vi "sv_Waterfall Display for Octave.vi"() -> ()   [LabVIEW 2017]
uses:
  <vilib>/addons/Sound and Vibration/compatibility/Waterfall/subVIs/sv_Waterfall for Octave Global.vi
panel:
  in  "palette":T1={"x axis width [%]"=80.0, "z axis height [%]"=40.0, "autoscale x"=FALSE, "autoscale y"=FALSE, "autoscale z max"=FALSE, "autoscale all"=FALSE, "transparency"=FALSE, "store view"=FALSE, "restore view"=FALSE} {"x axis width [%]" min=10.0 max=100.0 step=1.0 scale=10.0..100.0 scale format="%.1f"; "z axis height [%]" min=10.0 max=99.99 step=1.0 scale=10.0..100.0 scale format="%.1f"}
  in  "stop":bool
  in  "y axis":dbl(slide)=1234.0 scale=0.0..2.0 scale format="%.1f"
  in  "z axis":dbl(slide) scale=0.0..90.0 scale format="%.1f"
  in  "x axis":dbl(slide) scale=10.0..10000.0 scale format="%.1f"
  out "Graph":cluster{dbl[], dbl[]}[](graph)
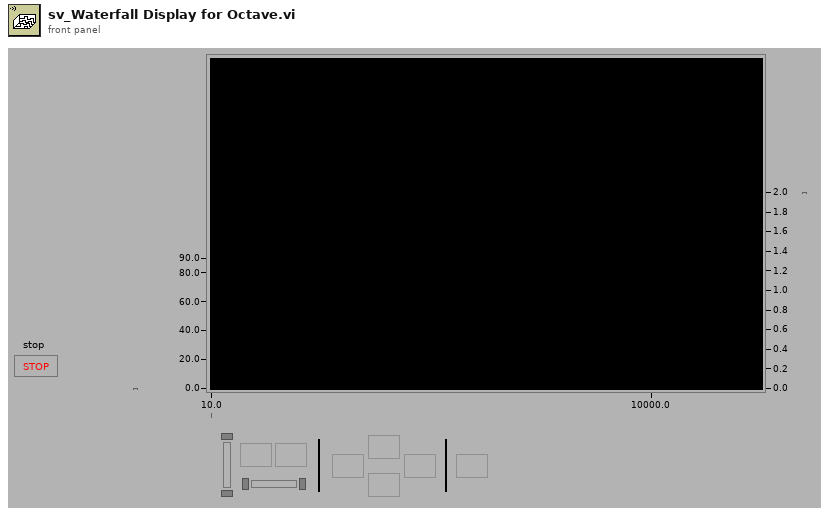
[diagram p1: front panel]
types:
  T1 = cluster{"x axis width [%]":dbl, "z axis height [%]":dbl, "autoscale x":bool, "autoscale y":bool, "autoscale z max":bool, "autoscale all":bool, "transparency":bool, "store view":bool, "restore view":bool}
  T2 = cluster{"autoscale x":bool, "autoscale y":bool, "autoscale z":bool, "autoscale all":bool, "transparency":bool, "store view":bool, "restore view":bool}
  T3 = cluster{"x axis width [%]":dbl, "z axis height [%]":dbl, "x axis minimum":dbl, "x axis maximum":dbl, "z axis minimum":dbl, "z axis maximum":dbl, "y axis minimum":dbl, "y axis maximum":dbl}
  T4 = typedef "LVPositionTypeDef.ctl" = cluster{"Left":i32, "Top":i32}
  T5 = cluster{"f low":dbl, "f high":dbl, "midband":dbl}[]
  T6 = cluster{"x axis width [%]":dbl, "z axis height [%]":dbl, "Scale.Minimum":dbl, "Scale.Maximum":dbl, "Scale.Minimum":dbl, "Scale.Maximum":dbl, "Scale.Minimum":dbl, "Scale.Maximum":dbl}
  T7 = cluster{"autoscale x":bool, "autoscale y":bool, "autoscale z max":bool, "autoscale all":bool, "transparency":bool, "store view":bool, "restore view":bool}
  T8 = cluster{"x axis width [%]":bool, "z axis height [%]":bool, bool, bool, bool, bool, bool, bool}
  T9 = cluster{"autoscale x":bool, "autoscale y":bool, bool, "autoscale all":bool, "transparency":bool, "store view":bool, "restore view":bool}
  T10 = cluster{bool, "x axis width [%]":dbl, "z axis height [%]":dbl, "Scale.Minimum":dbl, "Scale.Maximum":dbl, "Scale.Minimum":dbl, "Scale.Maximum":dbl, "Scale.Minimum":dbl, "Scale.Maximum":dbl, "transparency":bool}
  T11 = cluster{"x axis":string, "y axis":string, "z axis":string}
  T12 = cluster{"Scale.Minimum":dbl, "Scale.Maximum":dbl}
  T13 = cluster{"y index":i32, "y length":i32, "x index":i32, "x length":i32}
  T14 = cluster{"frame":u32, "plot":u32, "background":u32}
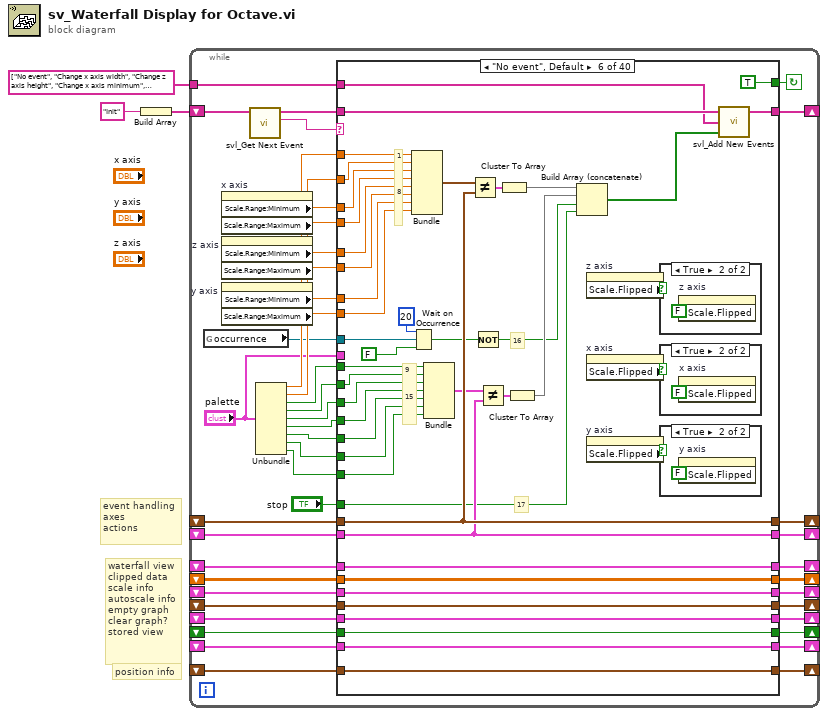
[diagram p0: block diagram]
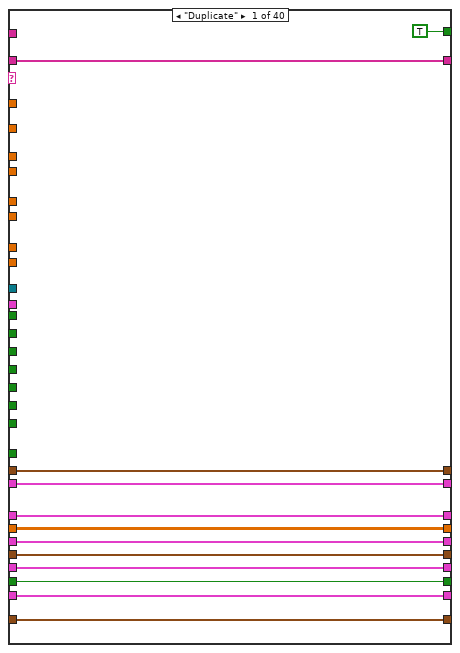
[diagram p2: hidden frame]
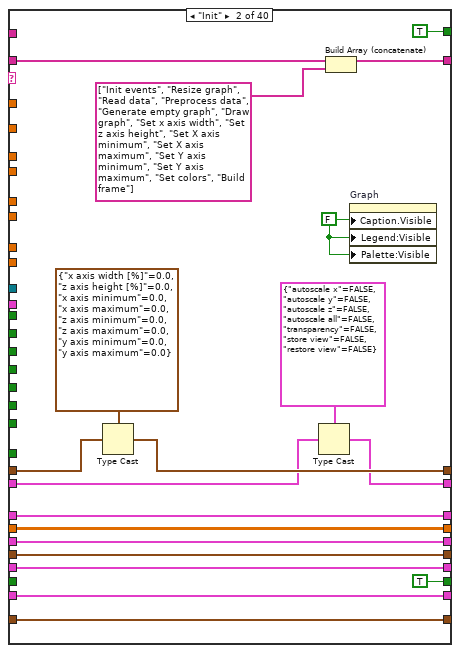
[diagram p3: hidden frame]
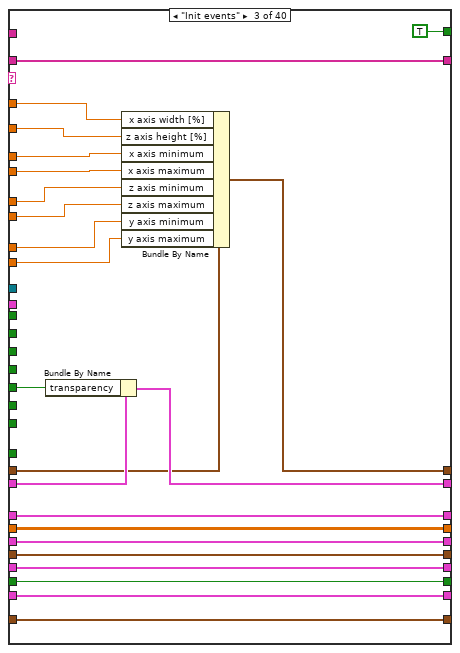
[diagram p4: hidden frame]
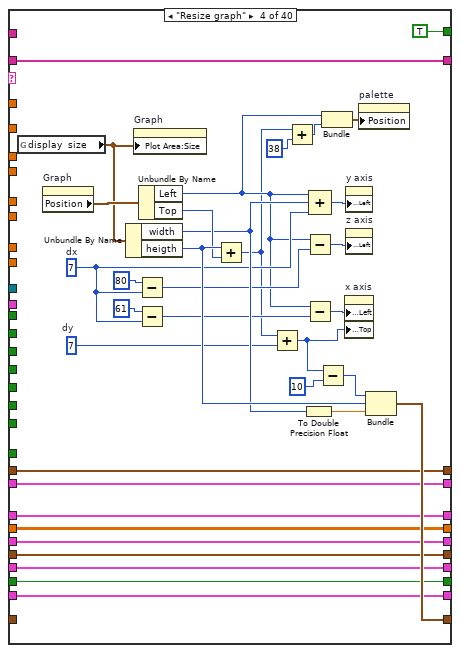
[diagram p5: hidden frame]
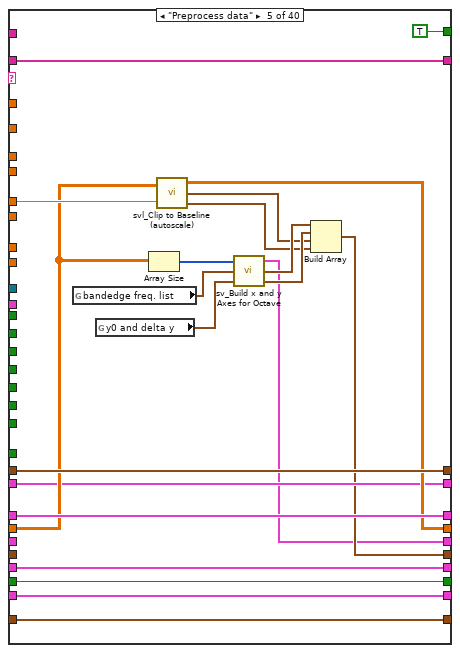
[diagram p6: hidden frame]
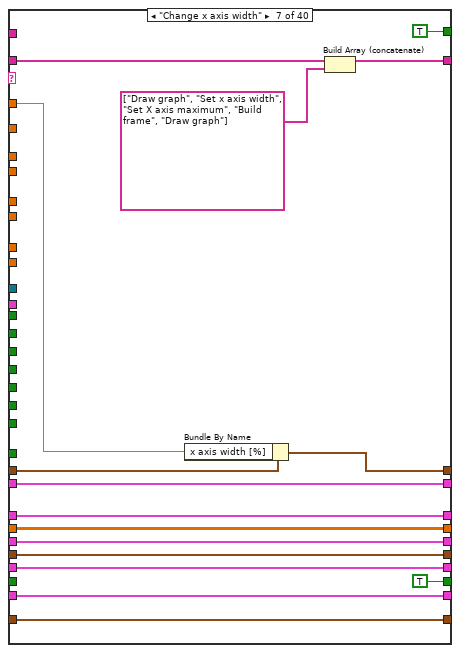
[diagram p10: hidden frame]
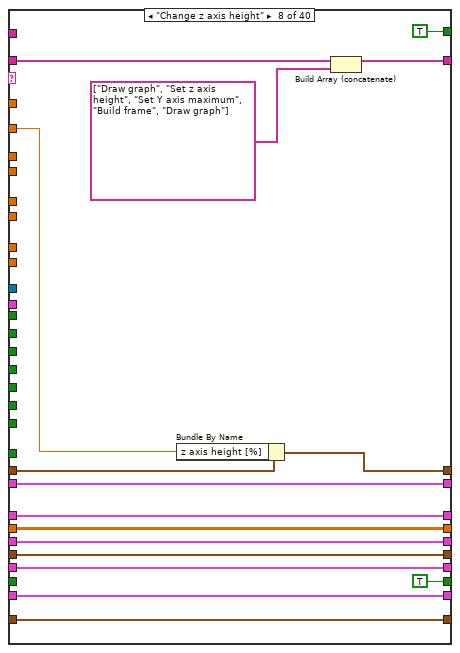
[diagram p11: hidden frame]
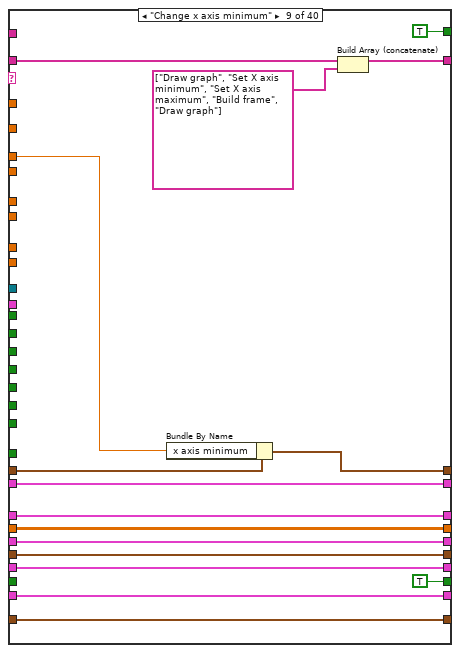
[diagram p12: hidden frame]
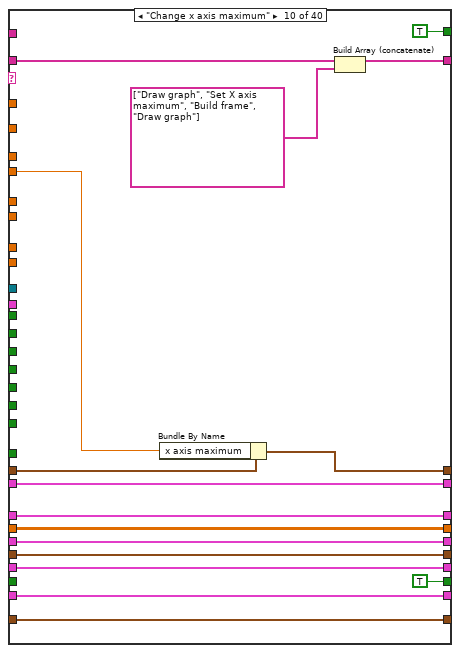
[diagram p13: hidden frame]
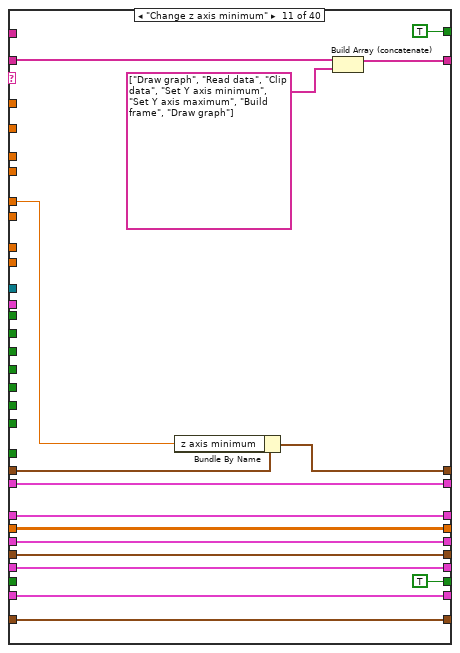
[diagram p14: hidden frame]
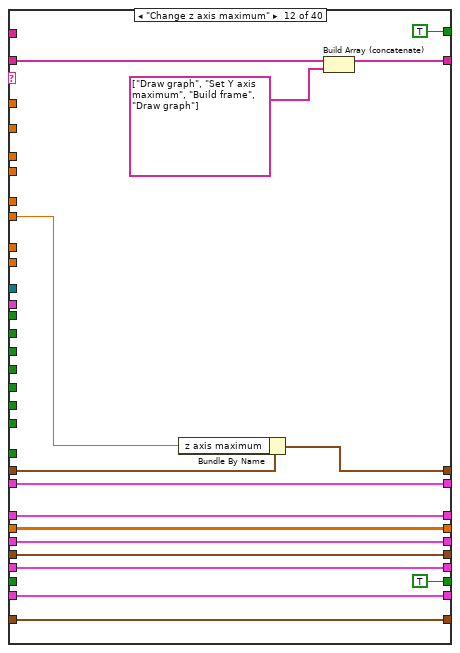
[diagram p15: hidden frame]
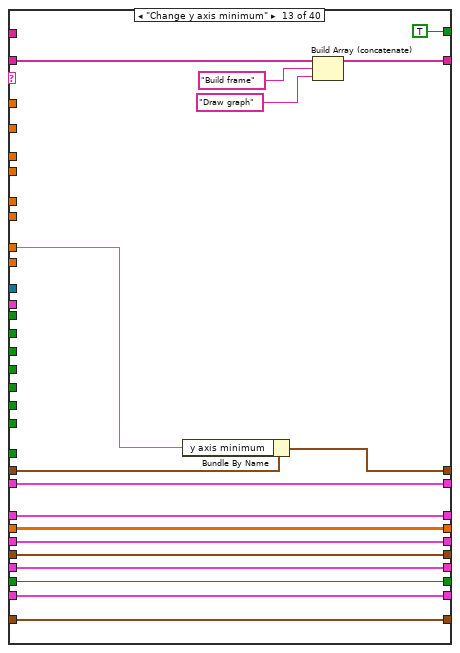
[diagram p16: hidden frame]
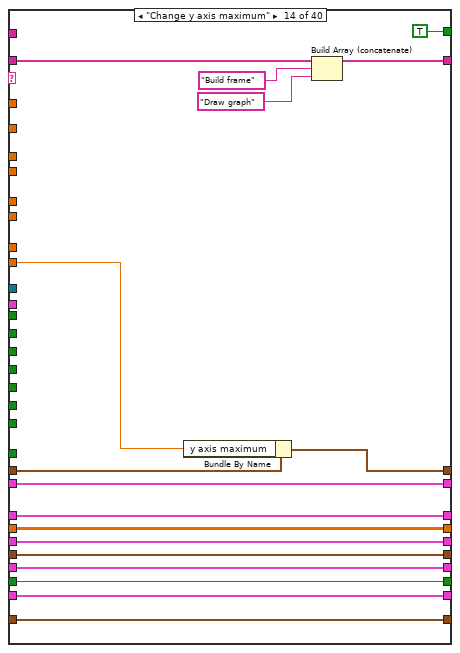
[diagram p17: hidden frame]
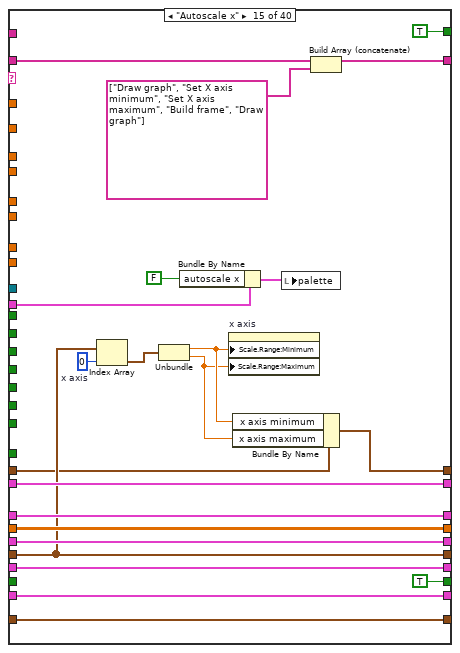
[diagram p18: hidden frame]
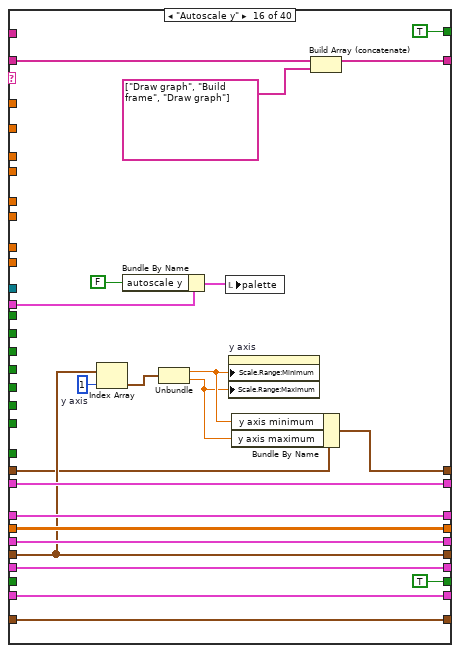
[diagram p19: hidden frame]
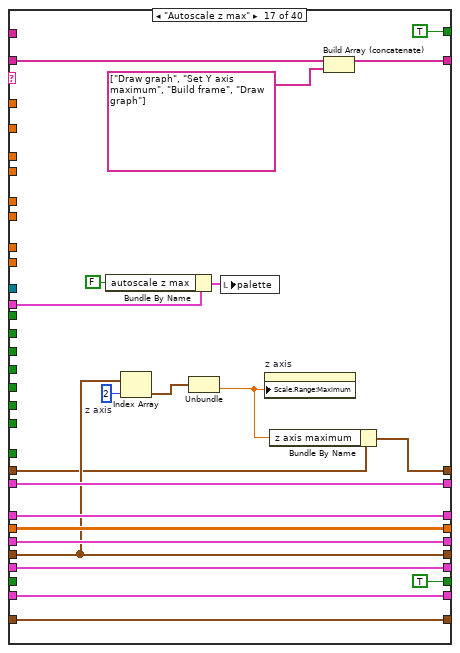
[diagram p20: hidden frame]
diagram:
  # "waterfall view\nclipped data\nscale info\nautoscale info\nempty graph\nclear graph?\nstored view"
  # "position info"
  # "event handling\naxes\nactions"
  n1 = Build Array("Init") -> (w2:string[])
  n2 = while {
    shift-left: _ -> [w16]
    shift-right: [w17] -> _
    shift-left: _ -> [w23]
    shift-right: [w22] -> _
    shift-left: _ -> [w25]
    shift-right: [w24] -> _
    shift-left: _ -> [w26]
    shift-right: [w27] -> _
    shift-left: _ -> [w29]
    shift-right: [w30] -> _
    shift-left: _ -> [w19]
    shift-right: [w32] -> _
    shift-left: _ -> [w31]
    shift-right: [w33] -> _
    shift-left: _ -> [w34]
    shift-right: [w35] -> _
    shift-left: _ -> [w38]
    shift-right: [w37] -> _
    shift-left: _ -> [w43]
    shift-right: [w44] -> _
    tunnel: string[] ["No event", "Change x axis width", "Change z axis height", "Change x axis minimum", "Change x axis maximum", "Change z axis minimum", "Change z axis maximum", "Change y axis minimum", "Change y axis maximum", "Autoscale x", "Autoscale y", "Autoscale z max", "Autoscale all", "Change transparency", "Store view", "Restore view", "Refresh", "Stop"] ("Event Names") -> [w46]
    shift-left: w2 -> [w21]
    shift-right: [w47] -> _
    stop <- w45 continue-if-true
    n3 = global read "sv_Waterfall for Octave Global.vi" "occurrence"() -> (w5:refnum<k4>)
    n4 = property on="x axis" class="Slide (strict)"() -> ("Scale.Range:Minimum"=w42:dbl, "Scale.Range:Maximum"=w41:dbl)  [unwired: 2 in, 2 out]
    n5 = property on="z axis" class="Slide (strict)"() -> ("Scale.Range:Minimum"=w40:dbl, "Scale.Range:Maximum"=w39:dbl)  [unwired: 2 in, 2 out]
    n6 = property on="y axis" class="Slide (strict)"() -> ("Scale.Range:Minimum"=w36:dbl, "Scale.Range:Maximum"=w28:dbl)  [unwired: 2 in, 2 out]
    n7 = call <vilib>:"svl_Get Next Event.vi"("Event Queue In"=w21) -> ("Next Event"=w4:string, "Event Queue Out"=w20:string[])  [unwired: 5 in]
    n8 = Unbundle("palette") -> ("x axis width [%]"=w15:dbl, "z axis height [%]"=w14:dbl, "autoscale x"=w7:bool, "autoscale y"=w8:bool, "autoscale z max"=w9:bool, "autoscale all"=w10:bool, "transparency"=w11:bool, "store view"=w12:bool, "restore view"=w13:bool)
    n9 = case shown="\"No event\", Default" w4 {
      tunnel: w20 -> [w58 w77 w93 w115 w156 w202 w220 w236 w251 w267 w283 w299 w307 w323 w345 w367 w387 w408 w424 w457 w465 w507 w528 w536 w572 w590 w630 w633 w653 w669 w683 w713 w735 w753 w757 w800 w808 w837 w865 w895]
      tunnel: [w58 w76 w93 w115 w156 w201 w219 w222 w250 w254 w282 w298 w308 w324 w346 w358 w388 w409 w423 w457 w466 w506 w528 w536 w572 w590 w630 w633 w653 w669 w683 w713 w735 w753 w757 w800 w808 w837 w865 w895] -> w47
      tunnel: w46 -> [_ _ _ _ _ w199 _ _ _ _ _ _ _ _ _ _ _ _ _ _ _ _ _ _ _ _ _ _ _ _ _ _ _ _ _ _ _ _ _ _]
      tunnel: [TRUE TRUE TRUE TRUE TRUE TRUE TRUE TRUE TRUE TRUE TRUE TRUE TRUE TRUE TRUE TRUE TRUE TRUE TRUE TRUE TRUE TRUE FALSE TRUE TRUE TRUE TRUE TRUE TRUE TRUE TRUE TRUE TRUE TRUE TRUE TRUE TRUE TRUE TRUE TRUE] -> w45
      tunnel: [w57 w72 w100 w125 w155 w197 w209 w225 w252 w268 w284 w300 w317 w334 w356 w378 w399 w416 w432 w456 w482 w515 w526 w558 w585 w601 w629 w644 w666 w680 w701 w712 w734 w752 w786 w799 w819 w848 w871 w894] -> w44
      tunnel: w43 -> [w57 w72 w100 _ w155 w197 w209 w225 w252 w268 w284 w300 w317 w334 w356 w378 w399 w416 w432 w456 w482 w515 w526 w558 w585 w601 w629 w644 w666 w680 w701 w712 w734 w752 w786 w799 w819 w848 w871 w894]
      tunnel: w15 -> [_ _ w84 _ _ w189 w210 _ _ _ _ _ _ _ _ _ _ _ _ w447 _ _ _ _ w580 _ _ _ w665 _ _ _ _ _ _ _ _ _ _ _]
      tunnel: w14 -> [_ _ w85 _ _ w196 _ w226 _ _ _ _ _ _ _ _ _ _ _ w446 _ _ _ _ _ w600 _ _ _ _ w694 _ _ _ w762 _ _ _ _ _]
      tunnel: w42 -> [_ _ w90 _ _ w195 _ _ w241 _ _ _ _ _ _ _ _ _ _ w445 _ _ _ _ _ _ _ w635 w650 _ _ _ _ _ w765 _ _ _ _ _]
      tunnel: w41 -> [_ _ w91 _ _ w190 _ _ _ w258 _ _ _ _ _ _ _ _ _ w444 _ _ _ _ _ _ _ _ w651 _ _ _ _ _ w760 _ _ _ _ _]
      tunnel: w40 -> [_ _ w89 _ w152 w194 _ _ _ _ w273 _ _ _ _ _ _ _ _ w443 _ _ _ _ _ _ _ _ _ w677 w693 _ w718 _ w758 _ _ _ _ _]
      tunnel: w39 -> [_ _ w88 _ _ w193 _ _ _ _ _ w291 _ _ _ _ _ _ _ w442 _ _ _ _ _ _ _ _ _ _ w692 _ _ _ w764 _ _ _ _ _]
      tunnel: [w56 w74 w80 w117 w154 w187 w218 w234 w242 w259 w276 w288 w309 w326 w344 w366 w390 w405 w431 w455 w481 w504 w525 w550 w581 w598 w620 w642 w662 w678 w684 w711 w727 w751 w784 w798 w818 w847 w870 w893] -> w37
      tunnel: w38 -> [w56 w73 w81 w117 w154 w187 w217 w235 w243 w260 w275 w289 w310 w327 w343 w365 w389 w405 w431 w455 w481 w503 w525 w549 w579 w599 w620 w643 w661 w679 w684 w711 w726 w751 w784 w798 w818 w847 w870 w893]
      tunnel: w36 -> [_ _ w87 _ _ w186 _ _ _ _ _ _ w304 _ _ _ _ _ _ w441 _ _ _ _ _ _ _ _ _ _ _ _ _ _ w773 _ _ _ _ _]
      tunnel: [w55 w71 w99 w116 w153 w184 w216 w233 w249 w266 w281 w297 w316 w333 w355 w377 w398 w415 w430 w454 w480 w514 w524 w557 w578 w597 w628 w641 w660 w676 w691 w710 w733 w750 w783 w793 w805 w834 w863 w892] -> w35
      tunnel: w34 -> [w55 w71 w99 w116 w153 w184 w216 w233 w249 w266 w281 w297 w316 w333 w355 w377 w398 w415 w430 w454 w480 w514 w524 w557 w578 w597 w628 w641 w660 w676 w691 w710 w733 w750 _ w793 w805 w834 w863 w892]
      tunnel: [w54 w70 w98 w114 w148 w183 w215 w232 w248 w265 w280 w296 w315 w332 w354 w376 w397 w414 w429 w453 w479 w513 w523 w556 w577 w596 w627 w640 w659 w675 w690 w703 w728 w740 w781 w797 w817 w846 w859 w891] -> w33
      tunnel: [w53 w69 w97 w113 w143 w182 w214 w231 w247 w264 w272 w295 w314 w331 w350 w372 w393 w406 w428 w452 w478 w512 w522 w540 w576 w595 w626 w639 w658 w674 w689 w707 w716 w744 w782 w796 w816 w845 w869 w890] -> w32
      tunnel: w31 -> [w54 w70 w98 w114 w145 w183 w215 w232 w248 w265 w280 w296 w315 w332 w354 w376 w397 w414 w429 w453 w479 w513 w523 w556 w577 w596 w627 w640 w659 w675 w690 _ w731 w740 w781 w797 w817 w846 w859 w891]
      tunnel: w19 -> [w53 w69 w97 w113 _ w182 w214 w231 w247 w264 w272 w295 w314 w331 w350 w372 w393 w406 w428 w452 w478 w512 w522 w540 w576 w595 w626 w639 w658 w674 w689 w707 w717 w744 w782 w796 w816 w845 w869 w890]
      tunnel: [w52 w68 w96 w112 w142 w181 w213 w230 w246 w263 w279 w294 w313 w330 w353 w375 w396 w413 w427 w451 w477 w511 w521 w555 w575 w594 w625 w638 w657 w673 w688 w706 w730 w745 w776 w795 w815 w844 w868 w889] -> w30
      tunnel: w29 -> [w52 w68 w96 w112 _ w181 w213 w230 w246 w263 w279 w294 w313 w330 w353 w375 w396 w413 w427 w451 w477 w511 w521 w555 w575 w594 w625 w638 w657 w673 w688 w706 w730 w745 w776 w795 w815 w844 w868 w889]
      tunnel: w28 -> [_ _ w86 _ _ w185 _ _ _ _ _ _ _ w325 _ _ _ _ _ w440 _ _ _ _ _ _ _ _ _ _ _ _ _ _ w774 _ _ _ _ _]
      tunnel: [w51 w67 w95 w111 w139 w180 w212 w229 w245 w262 w278 w293 w312 w329 w352 w374 w395 w412 w426 w450 w476 w510 w520 w554 w574 w593 w624 w637 w656 w672 w687 w708 w729 w749 w778 w794 w804 w833 w862 w888] -> w27
      tunnel: w26 -> [w51 w67 w95 w111 w139 w180 w212 w229 w245 w262 w278 w293 w312 w329 w352 w374 w395 w412 w426 w450 w476 w510 w520 w554 w574 w593 w624 w637 w656 w672 w687 w708 w729 _ w778 w794 w804 w833 w862 w888]
      tunnel: w25 -> [w50 _ w94 w110 w146 w179 _ _ _ _ _ _ w311 w328 _ _ _ _ _ w449 _ _ w519 w537 w571 w591 w623 w636 w655 w671 w686 w709 w732 w748 _ w790 w814 w843 w867 w887]
      tunnel: [w50 TRUE w94 w110 w146 w179 TRUE TRUE TRUE TRUE TRUE TRUE w311 w328 TRUE TRUE TRUE TRUE TRUE w449 TRUE w505 w519 w537 w571 w591 w623 w636 w655 w671 w686 w709 w732 w748 FALSE FALSE w814 w843 w867 w887] -> w24
      tunnel: w11 -> [_ _ w92 _ _ w174 _ _ _ _ _ _ _ _ _ _ _ _ w422 w439 _ _ _ _ _ _ _ _ _ _ _ _ _ _ _ _ w809 w838 _ _]
      tunnel: w23 -> [w49 w65 w83 w109 w144 w170 w211 w227 w240 w257 w274 w290 w306 w322 w351 w373 w394 w411 w421 w448 w475 w509 w518 w553 w573 w592 w622 w634 w654 w670 w685 w705 w725 w747 w770 w789 w810 w839 w866 w886]
      tunnel: [w49 w66 w82 w109 w144 w170 w211 w227 w240 w257 w274 w290 w306 w322 w351 w373 w394 w411 w420 w448 w475 w509 w518 w553 w573 w592 w622 w634 w654 w670 w685 w705 w725 w747 w770 w789 w810 w839 w866 w886] -> w22
      tunnel: w7 -> [_ _ _ _ _ w178 _ _ _ _ _ _ _ _ _ _ _ _ _ _ _ _ _ _ _ _ _ _ _ _ _ _ _ _ _ _ _ _ _ _]
      tunnel: w8 -> [_ _ _ _ _ w177 _ _ _ _ _ _ _ _ _ _ _ _ _ _ _ _ _ _ _ _ _ _ _ _ _ _ _ _ _ _ _ _ _ _]
      tunnel: w9 -> [_ _ _ _ _ w176 _ _ _ _ _ _ _ _ _ _ _ _ _ _ _ _ _ _ _ _ _ _ _ _ _ _ _ _ _ _ _ _ _ _]
      tunnel: w10 -> [_ _ _ _ _ w175 _ _ _ _ _ _ _ _ _ _ _ _ _ _ _ _ _ _ _ _ _ _ _ _ _ _ _ _ _ _ _ _ _ _]
      tunnel: "stop" -> [_ _ _ _ _ w163 _ _ _ _ _ _ _ _ _ _ _ _ _ _ _ _ _ _ _ _ _ _ _ _ _ _ _ _ _ _ _ _ _ _]
      tunnel: w12 -> [_ _ _ _ _ w169 _ _ _ _ _ _ _ _ _ _ _ _ _ _ _ _ _ _ _ _ _ _ _ _ _ _ _ _ _ _ _ _ _ _]
      tunnel: w13 -> [_ _ _ _ _ w168 _ _ _ _ _ _ _ _ _ _ _ _ _ _ _ _ _ _ _ _ _ _ _ _ _ _ _ _ _ _ _ _ _ _]
      tunnel: [w48 w62 w79 w108 w140 w167 w207 w224 w239 w256 w271 w287 w305 w321 w340 w362 w384 w407 w419 w438 w474 w508 w517 w538 w570 w589 w621 w632 w652 w668 w682 w704 w715 w746 w769 w788 w807 w836 w864 w885] -> w17
      tunnel: w16 -> [w48 w62 w79 w108 w140 w167 w207 w224 w239 w256 w271 w287 w305 w321 w340 w362 w384 w407 w419 _ w474 w508 w517 w538 w570 w589 w621 w632 w652 w668 w682 w704 w715 w746 w769 w788 w807 w836 w864 w885]
      tunnel: w5 -> [_ _ _ _ _ w160 _ _ _ _ _ _ _ _ _ _ _ _ _ _ _ _ _ _ _ _ _ _ _ _ _ _ _ _ _ _ _ _ _ _]
      tunnel: "palette" -> [_ _ _ _ _ _ _ _ _ _ _ _ _ _ w338 w359 w381 w402 _ w435 w464 _ _ _ _ _ _ _ _ _ _ _ _ _ _ _ _ _ _ _]
      frame "Duplicate" {
      }
      frame "Init" {
        w61 = FALSE ("Caption Visible")
        n10 = Type Cast(type=T3 {"x axis width [%]"=0.0, "z axis height [%]"=0.0, "x axis minimum"=0.0, "x axis maximum"=0.0, "z axis minimum"=0.0, "z axis maximum"=0.0, "y axis minimum"=0.0, "y axis maximum"=0.0}, x=w73) -> (*(type *) &x=w74:T3)
        n11 = Type Cast(type=T2 {"autoscale x"=FALSE, "autoscale y"=FALSE, "autoscale z"=FALSE, "autoscale all"=FALSE, "transparency"=FALSE, "store view"=FALSE, "restore view"=FALSE}, x=w65) -> (*(type *) &x=w66:T2)
        n12 = Build Array (concatenate)(w77, string[] ["Init events", "Resize graph", "Read data", "Preprocess data", "Generate empty graph", "Draw graph", "Set x axis width", "Set z axis height", "Set X axis minimum", "Set X axis maximum", "Set Y axis minimum", "Set Y axis maximum", "Set colors", "Build frame"]) -> (w76:string[])
        n13 = property on="Graph" class="XYGraph (strict)"("Caption.Visible"=w61, "Legend:Visible"=w61, "Palette:Visible"=w61) -> ()  [unwired: 2 in, 2 out]
      }
      frame "Init events" {
        n14 = Bundle By Name(cluster=w83, "transparency"=w92) -> (w82:T2)
        n15 = Bundle By Name(cluster=w81, "x axis width [%]"=w84, "z axis height [%]"=w85, "x axis minimum"=w90, "x axis maximum"=w91, "z axis minimum"=w89, "z axis maximum"=w88, "y axis minimum"=w87, "y axis maximum"=w86) -> (w80:T3)
      }
      frame "Resize graph" {
        w119 = u32 7  # dx
        w118 = u32 7  # dy
        n16 = global read "sv_Waterfall for Octave Global.vi" "display  size"() -> (w102:cluster{"width":u32, "heigth":u32})
        n17 = property on="Graph" class="XYGraph (strict)"() -> ("Position"=w126:T4)  [unwired: 2 in, 2 out]
        n18 = Unbundle By Name(w102) -> ("width"=w130:u32, "heigth"=w135:u32)
        n19 = property on="Graph" class="XYGraph (strict)"("Plot Area:Size"=w102) -> ()  [unwired: 2 in, 2 out]
        n20 = Subtract(x=u32 80, y=w119) -> (x-y=w123:u32)
        n21 = Subtract(x=u32 61, y=w119) -> (x-y=w121:u32)
        n22 = Unbundle By Name(w126) -> ("Left"=w106:i32, "Top"=w132:i32)
        n23 = Add(x=w135, y=w132) -> (x+y=w105:u32)
        n24 = Add(x=w105, y=w118) -> (x+y=w120:u32)
        n25 = Add(x=w105, y=u32 38) -> (x+y=w103:u32)
        n26 = To Double Precision Float(number=w130) -> (double precision float=w134:dbl)
        n27 = Subtract(x=w106, y=w123) -> (x-y=w129:u32)
        n28 = Subtract(x=w106, y=w121) -> (x-y=w127:u32)
        n29 = Compound Arithmetic op=ADD(w106, w130, w119) -> (w128:u32)
        n30 = Subtract(x=w120, y=u32 10) -> (x-y=w133:u32)
        n31 = Bundle("Left"=w106, w103) -> (w107:cluster{"Left":i32, u32})  [unwired: 1 in]
        n32 = property on="x axis" class="Slide (strict)"("Position:Left"=w127, "Position:Top"=w120) -> ()  [unwired: 2 in, 2 out]
        n33 = property on="y axis" class="Slide (strict)"("Position:Left"=w128) -> ()  [unwired: 2 in, 2 out]
        n34 = property on="z axis" class="Slide (strict)"("Position:Left"=w129) -> ()  [unwired: 2 in, 2 out]
        n35 = property on="palette" class="Clust (strict)"("Position"=w107) -> ()  [unwired: 2 in, 2 out]
        n36 = Bundle(w133, "heigth"=w135, w134) -> (w125:cluster{u32, "heigth":u32, dbl})  [unwired: 1 in]
      }
      frame "Preprocess data" {
        n37 = global read "sv_Waterfall for Octave Global.vi" "bandedge freq. list"() -> (w137:T5)
        n38 = global read "sv_Waterfall for Octave Global.vi" "y0 and delta y"() -> (w138:cluster{"y0":dbl, "delta y":dbl})
        n39 = Array Size(array=w145) -> (size(s)=w147:i32[])
        n40 = call <vilib>:"svl_Clip to Baseline (autoscale).vi"("waterfall data"=w145, "baseline"=w152) -> ("clipped data"=w148:dbl[][], "z autoscale"=w149:cluster{"z min":dbl, "z max":dbl}, "z scale"=w141:cluster{"z min":dbl, "z max":dbl})
        n41 = call <vilib>:"sv_Build x and y Axes for Octave.vi"("y0 and delta y"=w138, "bandedge freq. list"=w137, "size(s)"=w147) -> ("y autoscale"=w150:cluster{"y min":dbl, "y max":dbl}, "x autoscale"=w151:cluster{"x min":dbl, "x max":dbl}, "scale info"=w142:cluster{"x scale":dbl[], "y scale":dbl[]})
        n42 = Build Array(w151, w150, w149, w141) -> (w143:cluster{"z min":dbl, "z max":dbl}[])
      }
      frame "No event", Default {
        # "16"
        # "17"
        # "9\n   \n\n15"
        # "1\n \n \n \n8"
        n43 = Wait on Occurrence(1:FALSE ("ignore previous (T)"), 2:w160, 3:20 ("ms timeout (-1)")) -> (0:w158:bool)
        n44 = Bundle("x axis width [%]"=w189, "z axis height [%]"=w196, "Scale.Minimum"=w195, "Scale.Maximum"=w190, "Scale.Minimum"=w194, "Scale.Maximum"=w193, "Scale.Minimum"=w186, "Scale.Maximum"=w185) -> (w192:T6)  [unwired: 1 in]
        n45 = Bundle("autoscale x"=w178, "autoscale y"=w177, "autoscale z max"=w176, "autoscale all"=w175, "transparency"=w174, "store view"=w169, "restore view"=w168) -> (w171:T7)  [unwired: 1 in]
        n46 = Not Equal?(x=w192, y=w187) -> (x != y?=w191:T8)
        n47 = Not(x=w158) -> (.not. x?=w162:bool)
        n48 = Not Equal?(x=w171, y=w170) -> (x != y?=w173:T9)
        n49 = Cluster To Array(cluster=w191) -> (array=w188:bool[])
        n50 = Cluster To Array(cluster=w173) -> (array=w172:bool[])
        n51 = Build Array (concatenate)(w188, w172, w162, w163) -> (w200:bool[])
        n52 = property on="z axis" class="Slide (strict)"() -> ("Scale.Flipped"=w166:bool)  [unwired: 2 in, 2 out]
        n53 = property on="x axis" class="Slide (strict)"() -> ("Scale.Flipped"=w165:bool)  [unwired: 2 in, 2 out]
        n54 = property on="y axis" class="Slide (strict)"() -> ("Scale.Flipped"=w164:bool)  [unwired: 2 in, 2 out]
        n55 = case shown="True" w166 {
          frame False {
          }
          frame True {
            n56 = property on="z axis" class="Slide (strict)"("Scale.Flipped"=FALSE ("Flipped")) -> ()  [unwired: 2 in, 2 out]
          }
        }
        n57 = case shown="True" w165 {
          frame False {
          }
          frame True {
            n58 = property on="x axis" class="Slide (strict)"("Scale.Flipped"=FALSE ("Flipped")) -> ()  [unwired: 2 in, 2 out]
          }
        }
        n59 = case shown="True" w164 {
          frame False {
          }
          frame True {
            n60 = property on="y axis" class="Slide (strict)"("Scale.Flipped"=FALSE ("Flipped")) -> ()  [unwired: 2 in, 2 out]
          }
        }
        n61 = call <vilib>:"svl_Add New Events.vi"("New Events"=w200, "Event Names"=w199, "Event Queue In"=w202) -> ("Event Queue Out"=w201:string[])  [unwired: 2 in]
      }
      frame "Change x axis width" {
        n62 = Bundle By Name(cluster=w217, "x axis width [%]"=w210) -> (w218:T3)
        n63 = Build Array (concatenate)(w220, string[] ["Draw graph", "Set x axis width", "Set X axis maximum", "Build frame", "Draw graph"]) -> (w219:string[])
      }
      frame "Change z axis height" {
        n64 = Bundle By Name(cluster=w235, "z axis height [%]"=w226) -> (w234:T3)
        n65 = Build Array (concatenate)(w236, string[] ["Draw graph", "Set z axis height", "Set Y axis maximum", "Build frame", "Draw graph"]) -> (w222:string[])
      }
      frame "Change x axis minimum" {
        n66 = Bundle By Name(cluster=w243, "x axis minimum"=w241) -> (w242:T3)
        n67 = Build Array (concatenate)(w251, string[] ["Draw graph", "Set X axis minimum", "Set X axis maximum", "Build frame", "Draw graph"]) -> (w250:string[])
      }
      frame "Change x axis maximum" {
        n68 = Bundle By Name(cluster=w260, "x axis maximum"=w258) -> (w259:T3)
        n69 = Build Array (concatenate)(w267, string[] ["Draw graph", "Set X axis maximum", "Build frame", "Draw graph"]) -> (w254:string[])
      }
      frame "Change z axis minimum" {
        n70 = Bundle By Name(cluster=w275, "z axis minimum"=w273) -> (w276:T3)
        n71 = Build Array (concatenate)(w283, string[] ["Draw graph", "Read data", "Clip data", "Set Y axis minimum", "Set Y axis maximum", "Build frame", "Draw graph"]) -> (w282:string[])
      }
      frame "Change z axis maximum" {
        n72 = Bundle By Name(cluster=w289, "z axis maximum"=w291) -> (w288:T3)
        n73 = Build Array (concatenate)(w299, string[] ["Draw graph", "Set Y axis maximum", "Build frame", "Draw graph"]) -> (w298:string[])
      }
      frame "Change y axis minimum" {
        n74 = Bundle By Name(cluster=w310, "y axis minimum"=w304) -> (w309:T3)
        n75 = Build Array (concatenate)(w307, "Build frame", "Draw graph") -> (w308:string[])
      }
      frame "Change y axis maximum" {
        n76 = Bundle By Name(cluster=w327, "y axis maximum"=w325) -> (w326:T3)
        n77 = Build Array (concatenate)(w323, "Build frame", "Draw graph") -> (w324:string[])
      }
      frame "Autoscale x" {
        w349 = 0  # x axis
        n78 = Index Array(array=w350, index=w349) -> (element=w348:cluster{"z min":dbl, "z max":dbl})
        n79 = Unbundle(w348) -> ("z min"=w342:dbl, "z max"=w341:dbl)
        n80 = Bundle By Name(cluster=w338, "autoscale x"=FALSE) -> (w339:T1)
        n81 = property on="x axis" class="Slide (strict)"("Scale.Range:Minimum"=w342, "Scale.Range:Maximum"=w341) -> ()  [unwired: 2 in, 2 out]
        n82 = Bundle By Name(cluster=w343, "x axis minimum"=w342, "x axis maximum"=w341) -> (w344:T3)
        n83 = local write "palette"(w339) -> ()
        n84 = Build Array (concatenate)(w345, string[] ["Draw graph", "Set X axis minimum", "Set X axis maximum", "Build frame", "Draw graph"]) -> (w346:string[])
      }
      frame "Autoscale y" {
        w371 = 1  # y axis
        n85 = Index Array(array=w372, index=w371) -> (element=w370:cluster{"z min":dbl, "z max":dbl})
        n86 = Bundle By Name(cluster=w359, "autoscale y"=FALSE ("autoscale x")) -> (w361:T1)
        n87 = Unbundle(w370) -> ("z min"=w364:dbl, "z max"=w363:dbl)
        n88 = local write "palette"(w361) -> ()
        n89 = property on="y axis" class="Slide (strict)"("Scale.Range:Minimum"=w364, "Scale.Range:Maximum"=w363) -> ()  [unwired: 2 in, 2 out]
        n90 = Bundle By Name(cluster=w365, "y axis minimum"=w364, "y axis maximum"=w363) -> (w366:T3)
        n91 = Build Array (concatenate)(w367, string[] ["Draw graph", "Build frame", "Draw graph"]) -> (w358:string[])
      }
      frame "Autoscale z max" {
        w392 = 2  # z axis
        n92 = Bundle By Name(cluster=w381, "autoscale z max"=FALSE ("autoscale x")) -> (w383:T1)
        n93 = Index Array(array=w393, index=w392) -> (element=w386:cluster{"z min":dbl, "z max":dbl})
        n94 = Unbundle(w386) -> ("z max"=w385:dbl)  [unwired: 1 out]
        n95 = local write "palette"(w383) -> ()
        n96 = property on="z axis" class="Slide (strict)"("Scale.Range:Maximum"=w385) -> ()  [unwired: 2 in, 2 out]
        n97 = Bundle By Name(cluster=w389, "z axis maximum"=w385) -> (w390:T3)
        n98 = Build Array (concatenate)(w387, string[] ["Draw graph", "Set Y axis maximum", "Build frame", "Draw graph"]) -> (w388:string[])
      }
      frame "Autoscale all" {
        n99 = Bundle By Name(cluster=w402, "autoscale all"=FALSE ("autoscale x")) -> (w404:T1)
        n100 = local write "palette"(w404) -> ()
        n101 = Build Array (concatenate)(w408, string[] ["Draw graph", "Set all scales", "Set X axis minimum", "Set X axis maximum", "Set Y axis maximum", "Build frame", "Draw graph"]) -> (w409:string[])
      }
      frame "Change transparency" {
        n102 = Bundle By Name(cluster=w421, "transparency"=w422) -> (w420:T2)
        n103 = Build Array (concatenate)(w424, string[] ["Draw graph", "Set transparency", "Draw graph"]) -> (w423:string[])
      }
      frame "Store view" {
        n104 = Bundle By Name(cluster=w435, "store view"=FALSE ("autoscale x")) -> (w437:T1)
        n105 = Bundle(TRUE, "x axis width [%]"=w447, "z axis height [%]"=w446, "Scale.Minimum"=w445, "Scale.Maximum"=w444, "Scale.Minimum"=w443, "Scale.Maximum"=w442, "Scale.Minimum"=w441, "Scale.Maximum"=w440, "transparency"=w439) -> (w438:T10)  [unwired: 1 in]
        n106 = local write "palette"(w437) -> ()
      }
      frame "Restore view" {
        n107 = Unbundle(w474) -> (w460:bool, "x axis width [%]"=w463:dbl, "z axis height [%]"=w462:dbl, "Scale.Minimum"=w473:dbl, "Scale.Maximum"=w472:dbl, "Scale.Minimum"=w471:dbl, "Scale.Maximum"=w470:dbl, "Scale.Minimum"=w469:dbl, "Scale.Maximum"=w468:dbl, "transparency"=w461:bool)
        n108 = case shown="True" w460 {
          tunnel: w473 -> [_ w502]
          tunnel: w472 -> [_ w501]
          tunnel: w471 -> [_ w500]
          tunnel: w470 -> [_ w499]
          tunnel: w469 -> [_ w498]
          tunnel: w468 -> [_ w497]
          tunnel: [w487 w496] -> w466
          tunnel: w465 -> [w487 w495]
          tunnel: w464 -> [w485 w494]
          tunnel: w463 -> [_ w493]
          tunnel: w462 -> [_ w492]
          tunnel: w461 -> [_ w491]
          tunnel: [w486 w488] -> w459
          frame False {
            n109 = Bundle By Name(cluster=w485, "restore view"=FALSE) -> (w486:T1)
          }
          frame True {
            n110 = Bundle By Name(cluster=w494, "x axis width [%]"=w493, "z axis height [%]"=w492, "transparency"=w491, "restore view"=FALSE) -> (w488:T1)
            n111 = property on="x axis" class="Slide (strict)"("Scale.Range:Minimum"=w502, "Scale.Range:Maximum"=w501) -> ()  [unwired: 2 in, 2 out]
            n112 = property on="z axis" class="Slide (strict)"("Scale.Range:Minimum"=w500, "Scale.Range:Maximum"=w499) -> ()  [unwired: 2 in, 2 out]
            n113 = property on="y axis" class="Slide (strict)"("Scale.Range:Minimum"=w498, "Scale.Range:Maximum"=w497) -> ()  [unwired: 2 in, 2 out]
            n114 = Build Array (concatenate)(w495, string[] ["Draw graph", "Init events", "Read data", "Clip data", "Set x axis width", "Set z axis height", "Set X axis minimum", "Set X axis maximum", "Set Y axis minimum", "Set Y axis maximum", "Set transparency", "Build frame", "Draw graph"]) -> (w496:string[])
          }
        }
        n115 = local write "palette"(w459) -> ()
      }
      frame "Refresh" {
        n116 = call <vilib>:"sv_Refresh for Octave.vi"("axes IN"=w503, "event queue IN"=w507) -> ("clear graph?"=w505:bool, "axes OUT"=w504:T3, "event queue OUT"=w506:string[])  [unwired: 1 in]
      }
      frame "Stop" {
      }
      frame "Set all scales" {
        w529 = " "  # non-breaking space (Alt 0160)
        w542 = 2  # z axis
        w546 = 1  # y axis
        w552 = 0  # x axis
        n117 = Index Array(array=w540, index=w552) -> (element=w551:cluster{"z min":dbl, "z max":dbl})
        n118 = Index Array(array=w540, index=w542) -> (element=w541:cluster{"z min":dbl, "z max":dbl})
        n119 = Index Array(array=w540, index=w546) -> (element=w545:cluster{"z min":dbl, "z max":dbl})
        n120 = global read "sv_Waterfall for Octave Global.vi" "axis labels"() -> (w535:T11)
        n121 = Unbundle(w551) -> ("z min"=w548:dbl, "z max"=w547:dbl)
        n122 = Unbundle(w545) -> ("z min"=w544:dbl, "z max"=w543:dbl)
        n123 = Unbundle(w541) -> ("z max"=w539:dbl)  [unwired: 1 out]
        n124 = Unbundle(w535) -> ("x axis"=w534:string, "y axis"=w531:string, "z axis"=w530:string)
        n125 = Concatenate Strings(w531, w529) -> (w533:string)
        n126 = Concatenate Strings(w530, w529) -> (w532:string)
        n127 = stacked-sequence {
          tunnel: w548 -> [_ w569]
          tunnel: w547 -> [_ w568]
          tunnel: w544 -> [_ w567]
          tunnel: w543 -> [_ w566]
          tunnel: w539 -> [_ w565]
          tunnel: w534 -> [_ w564]
          tunnel: w532 -> [_ w563]
          tunnel: w533 -> [_ w562]
          frame #0 {
            w561 = refnum<vi> refnum  # Panel
            n128 = property class="Pnl"(reference=w561, "Defer Panel Updates"=TRUE) -> ()  [unwired: 1 in, 2 out]
          }
          frame #1 {
            n129 = property on="x axis" class="Slide (strict)"("Scale.Range:Minimum"=w569, "Scale.Range:Maximum"=w568, "Caption.Text"=w564) -> ()  [unwired: 2 in, 2 out]
            n130 = property on="y axis" class="Slide (strict)"("Scale.Range:Minimum"=w567, "Scale.Range:Maximum"=w566, "Caption.Text"=w562) -> ()  [unwired: 2 in, 2 out]
            n131 = property on="z axis" class="Slide (strict)"("Scale.Range:Maximum"=w565, "Caption.Text"=w563) -> ()  [unwired: 2 in, 2 out]
          }
        }
        n132 = Bundle By Name(cluster=w549, "z axis maximum"=w539, "y axis minimum"=w544, "y axis maximum"=w543, "x axis minimum"=w548, "x axis maximum"=w547) -> (w550:T3)
      }
      frame "Set x axis width" {
        n133 = Unbundle(w585) -> (w584:dbl)  [unwired: 2 out]
        n134 = Compound Arithmetic op=MULTIPLY(w580, w584, 0.01) -> (w586:dbl)
        n135 = Bundle By Name(cluster=w579, "x axis width [%]"=w580) -> (w581:T3)
        n136 = Round Toward +Infinity(x=w586) -> (ceil(x): smallest int >= x=w582:dbl)
        n137 = To Unsigned Long Integer(number=w582) -> (unsigned 32bit integer=w587:u32)
        n138 = property on="x axis" class="Slide (strict)"("Housing Size:Width"=w587) -> ()  [unwired: 2 in, 2 out]
      }
      frame "Set z axis height" {
        n139 = stacked-sequence {
          tunnel: w601 -> [_ _ w609 _]
          tunnel: w600 -> [_ _ w607 _]
          frame #0 {
            w604 = refnum<vi> refnum  # Panel
            n140 = property class="Pnl"(reference=w604, "Defer Panel Updates"=TRUE) -> ()  [unwired: 1 in, 2 out]
          }
          frame #1 {
            w605 = FALSE ("Caption.Visible")
            n141 = property on="y axis" class="Slide (strict)"("Caption.Visible"=w605) -> ()  [unwired: 2 in, 2 out]
            n142 = property on="z axis" class="Slide (strict)"("Caption.Visible"=w605) -> ()  [unwired: 2 in, 2 out]
          }
          frame #2 {
            n143 = Unbundle(w609) -> (w616:u32, "heigth"=w617:u32)  [unwired: 1 out]
            n144 = To Double Precision Float(number=w617) -> (double precision float=w615:dbl)
            n145 = Compound Arithmetic op=MULTIPLY(w607, w615, 0.01) -> (w610:dbl)
            n146 = Round Toward +Infinity(x=w610) -> (ceil(x): smallest int >= x=w608:dbl)
            n147 = To Unsigned Long Integer(number=w608) -> (unsigned 32bit integer=w612:u32)
            n148 = Subtract(x=w617, y=w612) -> (x-y=w613:u32)
            n149 = Subtract(x=w616, y=w613) -> (x-y=w614:u32)
            n150 = Subtract(x=w616, y=w612) -> (x-y=w611:u32)
            n151 = property on="z axis" class="Slide (strict)"("Position:Top"=w611, "Housing Size:Height"=w612) -> ()  [unwired: 2 in, 2 out]
            n152 = property on="y axis" class="Slide (strict)"("Position:Top"=w614, "Housing Size:Height"=w613) -> ()  [unwired: 2 in, 2 out]
          }
          frame #3 {
            w618 = TRUE ("Caption.Visible")
            n153 = property on="y axis" class="Slide (strict)"("Caption.Visible"=w618) -> ()  [unwired: 2 in, 2 out]
            n154 = property on="z axis" class="Slide (strict)"("Caption.Visible"=w618) -> ()  [unwired: 2 in, 2 out]
          }
        }
        n155 = Bundle By Name(cluster=w599, "z axis height [%]"=w600) -> (w598:T3)
      }
      frame "Set z axis minimum" {
        n156 = Unbundle By Name(w620) -> ("z axis minimum"=w619:dbl)
        n157 = property on="z axis" class="Slide (strict)"("Scale.Range:Minimum"=w619) -> ()  [unwired: 2 in, 2 out]
      }
      frame "Set X axis minimum" {
        n158 = property on="Graph" class="XYGraph (strict)"("X Scale.Range:Minimum"=w635) -> ()  [unwired: 2 in, 2 out]
        n159 = Bundle By Name(cluster=w643, "x axis minimum"=w635) -> (w642:T3)
      }
      frame "Set X axis maximum" {
        n160 = Multiply(x=0.01, y=w665) -> (x*y=w663:dbl)
        n161 = Divide(x=w651, y=w650) -> (x/y=w649:dbl)
        n162 = Reciprocal(x=w663) -> (1/x=w648:dbl)
        n163 = Power Of X(1:w649, 2:w648) -> (0:w647:dbl)
        n164 = Bundle By Name(cluster=w661, "x axis maximum"=w651) -> (w662:T3)
        n165 = Multiply(x=w647, y=w650) -> (x*y=w646:dbl)
        n166 = property on="Graph" class="XYGraph (strict)"("X Scale.Range:Maximum"=w646) -> ()  [unwired: 2 in, 2 out]
      }
      frame "Set Y axis minimum" {
        n167 = property on="Graph" class="XYGraph (strict)"("Y Scale.Range:Minimum"=w677) -> ()  [unwired: 2 in, 2 out]
        n168 = Bundle By Name(cluster=w679, "z axis minimum"=w677) -> (w678:T3)
      }
      frame "Set Y axis maximum" {
        n169 = Multiply(x=0.01, y=w694) -> (x*y=w698:dbl)
        n170 = Subtract(x=w692, y=w693) -> (x-y=w697:dbl)
        n171 = Reciprocal(x=w698) -> (1/x=w696:dbl)
        n172 = Multiply(x=w696, y=w697) -> (x*y=w695:dbl)
        n173 = Add(x=w695, y=w693) -> (x+y=w700:dbl)
        n174 = property on="Graph" class="XYGraph (strict)"("Y Scale.Range:Maximum"=w700) -> ()  [unwired: 2 in, 2 out]
      }
      frame "Read data" {
        n175 = global read "sv_Waterfall for Octave Global.vi" "waterfall data"() -> (w703:dbl[][])
      }
      frame "Clip data" {
        w724 = 3  # absolute z max
        w722 = 2  # z axis
        n176 = call <vilib>:"svl_Clip to Baseline.vi"("baseline"=w718, "waterfall data"=w731) -> ("clipped data"=w728:dbl[][])
        n177 = Index Array(array=w717, index=w724) -> (element=w723:cluster{"z min":dbl, "z max":dbl})
        n178 = Unbundle(w723) -> ("z max"=w721:dbl)  [unwired: 1 out]
        n179 = Bundle By Name(cluster=w726, "z axis minimum"=w718) -> (w727:T3)
        n180 = Bundle("Scale.Minimum"=w718, "z max"=w721) -> (w720:cluster{"Scale.Minimum":dbl, "z max":dbl})  [unwired: 1 in]
        n181 = call <vilib>:"svl_Autoscale.vi"("scale"=w720) -> ("autoscale"=w719:cluster{"min":dbl, "max":dbl})
        n182 = Replace Array Subset(array=w717, new element=w719, index=w722) -> (w716:cluster{"z min":dbl, "z max":dbl}[])
      }
      frame "Generate empty graph" {
        n183 = Array Size(array=w740) -> (size(s)=w739:i32[])
        n184 = Index Array(array=w739, index=0) -> (element=w737:i32)
        n185 = Add(x=w737, y=2) -> (x+y=w742:i32)
        n186 = Initialize Array(cluster{dbl[], dbl[]} {[nan], [nan]} ("frame"), w742) -> (w749:cluster{dbl[], dbl[]}[])
      }
      frame "Build frame" {
        w755 = refnum<vi> refnum  # Panel
        n187 = Bundle("Scale.Minimum"=w765, "Scale.Maximum"=w760) -> (w759:T12)  [unwired: 1 in]
        n188 = Bundle("Scale.Minimum"=w758, "Scale.Maximum"=w764) -> (w761:T12)  [unwired: 1 in]
        n189 = Bundle("Scale.Minimum"=w773, "Scale.Maximum"=w774) -> (w772:T12)  [unwired: 1 in]
        n190 = property on="Graph" class="XYGraph (strict)"() -> ("X Scale.Range:Maximum"=w763:dbl, "Y Scale.Range:Maximum"=w785:dbl)  [unwired: 2 in, 2 out]
        n191 = call <vilib>:"sv_Limit x and y Axes for Octave.vi"("y scale"=w772, "x scale"=w759, "scale info"=w776) -> ("subset info"=w771:T13, "scale subset"=w775:cluster{"x scale":dbl[], "y scale":dbl[]})
        n192 = call <vilib>:"sv_Compute Frame and Perspective for Octave.vi"("x scale"=w759, "z scale"=w761, "z axis height [%]"=w762, "X maximum"=w763, "Y maximum"=w785) -> ("front frame"=w766:cluster{dbl[], dbl[]}, "back frame"=w767:cluster{dbl[], dbl[]}, "dY"=w780:dbl, "dX"=w779:dbl)  [unwired: 2 in]
        n193 = property class="Pnl"(reference=w755, "Defer Panel Updates"=FALSE) -> ()  [unwired: 1 in, 2 out]
        n194 = call <vilib>:"sv_Generate Waterfall View for Octave.vi"("baseline"=w758, "scale info"=w775, "clipped data"=w781, "dX"=w779, "dY"=w780, "y scale"=w772, "subset info"=w771) -> ("waterfall view"=w768:cluster{dbl[], dbl[]}[])  [unwired: 4 in]
        n195 = Build Array (concatenate)(w766, w768, w767) -> (w783:cluster{dbl[], dbl[]}[])
      }
      frame "Draw graph" {
        n196 = Select(t=w794, s=w790, f=w793) -> (s? t:f=→"Graph":cluster{dbl[], dbl[]}[])
      }
      frame "Set transparency" {
        n197 = Array Size(array=w804) -> (size(s)=w806:i32)
        n198 = Decrement(x=w806) -> (x-1=w802:i32)
        n199 = Decrement(x=w802) -> (x-1=w803:i32)
        n200 = Select(t=i16 -1, s=w809, f=i16 -3 ("t")) -> (s? t:f=w811:i16)
        n201 = for {
          N: w803 -> [_]
          tunnel: w811 -> [w821]
          i -> [w823]
          n202 = Increment(x=w823) -> (x+1=w822:i32)
          n203 = property on="Graph" class="XYGraph (strict)"("Active Plot"=w822, "Plot.Fill To"=w821) -> ()  [unwired: 2 in, 2 out]
        }
      }
      frame "Set colors" {
        w832 = i16 -1 ("Fill To")
        n204 = global read "sv_Waterfall for Octave Global.vi" "colors"() -> (w825:T14)
        n205 = Array Size(array=w833) -> (size(s)=w835:i32)
        n206 = Unbundle By Name(w825) -> ("frame"=w828:u32)
        n207 = Unbundle By Name(w825) -> ("background"=w826:u32)
        n208 = Unbundle By Name(w825) -> ("plot"=w827:u32)
        n209 = Decrement(x=w835) -> (x-1=w831:i32)
        n210 = Select(t=i16 -1, s=w838, f=i16 -3 ("t")) -> (s? t:f=w840:i16)
        n211 = Decrement(x=w831) -> (x-1=w829:i32)
        n212 = for {
          N: w829 -> [_]
          tunnel: w826 -> [w855]
          tunnel: w840 -> [w854]
          tunnel: w827 -> [w851]
          i -> [w853]
          n213 = Increment(x=w853) -> (x+1=w852:i32)
          n214 = property on="Graph" class="XYGraph (strict)"("Active Plot"=w852, "Plot.Plot Color"=w851, "Plot.Fill/Point Color"=w855, "Plot.Fill To"=w854, "Plot.Plot Interpolation"=u8 3 ("Plot Interpolation")) -> ()  [unwired: 2 in, 2 out]
        }
        n215 = property on="Graph" class="XYGraph (strict)"("Plot Area:Colors:BG Color"=w826) -> ()  [unwired: 2 in, 2 out]
        n216 = property on="Graph" class="XYGraph (strict)"("Active Plot"=u32 0, "Plot.Plot Color"=w828, "Plot.Fill To"=w832, "Active Plot"=w831, "Plot.Plot Color"=w828, "Plot.Fill To"=w832, "Plot.Plot Interpolation"=u8 2 ("Plot Interpolation")) -> ()  [unwired: 2 in, 2 out]
      }
      frame "Refresh colors" {
        n217 = Array Size(array=w862) -> (size(s)=w857:i32)
        n218 = Array Size(array=w859) -> (size(s)=w860:i32[])
        n219 = Index Array(array=w860, index=0) -> (element=w858:i32)
        n220 = Not Equal?(x=w857, y=w858) -> (x != y?=w856:bool)
        n221 = case shown="True" w856 {
          tunnel: w857 -> [_ w879]
          frame False {
          }
          frame True {
            n222 = global read "sv_Waterfall for Octave Global.vi" "colors"() -> (w874:T14)
            n223 = Decrement(x=w879) -> (x-1=w878:i32)
            n224 = Unbundle By Name(w874) -> ("frame"=w876:u32, "plot"=w875:u32)
            n225 = Decrement(x=w878) -> (x-1=w877:i32)
            n226 = for {
              N: w877 -> [_]
              tunnel: w875 -> [w881]
              i -> [w883]
              n227 = Increment(x=w883) -> (x+1=w882:i32)
              n228 = property on="Graph" class="XYGraph (strict)"("Active Plot"=w882, "Plot.Plot Color"=w881, "Plot.Plot Interpolation"=u8 3 ("Plot Interpolation")) -> ()  [unwired: 2 in, 2 out]
            }
            n229 = property on="Graph" class="XYGraph (strict)"("Active Plot"=w878, "Plot.Plot Color"=w876, "Plot.Plot Interpolation"=u8 2 ("Plot Interpolation")) -> ()  [unwired: 2 in, 2 out]
          }
        }
      }
      frame "Open front panel" {
        n230 = global read "sv_Waterfall for Octave Global.vi" "frontmost (T)"() -> (w884:bool)
        n231 = case shown="True" w884 {
          frame False {
          }
          frame True {
            n232 = Open VI Reference(vi path="Waterfall Display for Octave.vi") -> (vi reference=w900:refnum<vi>)  [unwired: 5 in, 1 out]
            n233 = property class="VI"(reference=w900, "Front Panel Window:Open"=TRUE ("Front Panel.Open")) -> (reference out=w897:refnum<vi>)  [unwired: 1 in, 1 out]
            n234 = Close Reference(reference=w897) -> ()  [unwired: 1 in, 1 out]
          }
        }
      }
    }
  }
